vi "Configure Bias_.vi"(7 "DC Bias State (F:Disable)":bool, 8 "error in (no error)":errorcluster, 9 "DC Bias Type (0: Voltage)":u16(ring) items=["Voltage", "Current"], 10 "DC Bias Level (0.0 V)":dbl, 11 "Agilent E4980 in":refnum<class "Agilent E4980.lvclass">) -> (0 "error out":errorcluster, 3 "Agilent E4980 out":refnum<class "Agilent E4980.lvclass">)   [LabVIEW 2020, in "Agilent E4980.lvclass"]
uses:
  Agilent E4980.lvclass
  C:/Sandbox/RF Bench/Source Code/WiSpry Test Framework/Instruments/Instrument.lvclass
  Instrument.lvclass/Instrument.ctl
  Instrument.lvclass
  <instrlib>/Agilent E4980/Agilent E4980.lvlib
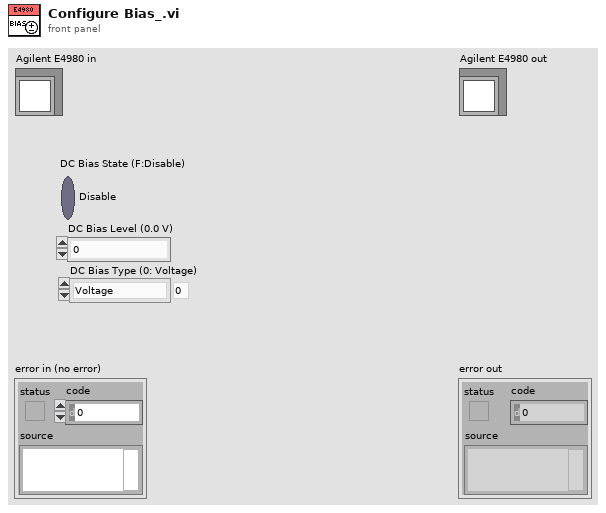
[diagram p1: front panel]
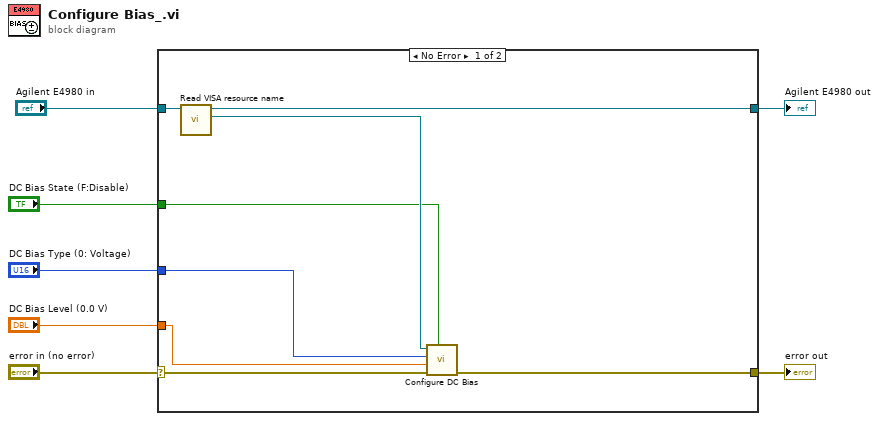
[diagram p0: block diagram]
diagram:
  n1 = case shown="No Error" "error in (no error)" {
    selector: "error in (no error)" -> [w9 w17]
    tunnel: [w8 w17] -> w7
    tunnel: [w14 w16] -> w6
    tunnel: "Agilent E4980 in" -> [w15 w16]
    tunnel: "DC Bias State (F:Disable)" -> [w12 _]
    tunnel: "DC Bias Level (0.0 V)" -> [w11 _]
    tunnel: "DC Bias Type (0: Voltage)" -> [w10 _]
    frame No Error {
      n2 = call "Read VISA resource name.vi"("Instrument in"=w15) -> ("VISA resource name"=w13:refnum<visa-resource-name>, "Instrument out"=w14:refnum<class "Agilent E4980.lvclass">)  [unwired: 9 in]
      n3 = call <instrlib>:"Configure DC Bias.vi"("DC Bias State (F:Disable)"=w12, "error in (no error)"=w9, "DC Bias Level (0.0 V)"=w11, "DC Bias Type (0: Voltage)"=w10, "VISA resource name"=w13) -> ("error out"=w8:errorcluster)  [unwired: 5 in, 1 out]
    }
    frame Error {
    }
  }
  "error out" <- w7
  "Agilent E4980 out" <- w6
